vi "Example Output - Char.vi"(11 "string":string) -> (3 "char":u16)   [LabVIEW 2010]
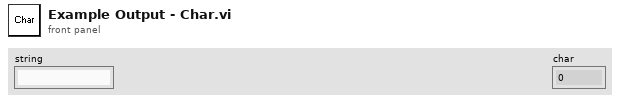
[diagram p1: front panel]
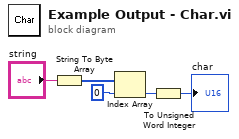
[diagram p0: block diagram]
diagram:
  n1 = String To Byte Array(string="string") -> (unsigned byte array=w4:u8[])
  n2 = Index Array(array=w4, index=0) -> (element=w2:u8)
  n3 = To Unsigned Word Integer(number=w2) -> (unsigned 16bit integer=→"char":u16)
